vi "PidHmiFloatToTwoWordsInArray.vi"(11 "Float":sgl) -> (3 "TwoWordArray":u16[](array[numeric]))   [LabVIEW 2018, in "Pid.lvlib"]
uses:
  Pid.lvlib
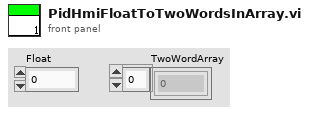
[diagram p1: front panel]
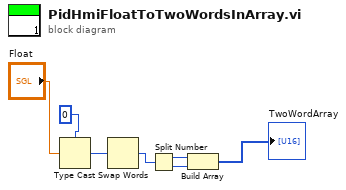
[diagram p0: block diagram]
diagram:
  n1 = Type Cast(type=u32 0 ("x"), x="Float") -> (*(type *) &x=w3:u32)
  n2 = Swap Words(1:w3) -> (0:w4:u32)
  n3 = Split Number(x=w4) -> (hi(x)=w5:u16, lo(x)=w6:u16)
  n4 = Build Array(w5, w6) -> (→"TwoWordArray":u16[])
